vi "checkout.vi"(0 "HGF_Reference":refnum<class "HGF_Reference.lvclass">, 3 "timeout in ms (-1)":i32=-1, 5 "error in (no error)":errorcluster) -> (14 "dup HGF_Reference":refnum<class "HGF_Reference.lvclass">, 16 "Object":refnum<class>, 17 "got object?":bool, 19 "error out":errorcluster)   [LabVIEW 2014, in "HGF_BaseClasses.lvlib" / "HGF_Reference.lvclass"]
doc: "Check out the referenced Object.\n\n<B>Attention:</B> Error in is ignored, but forwarded.\nDo not forget to check in again, if you have got the object."
uses:
  HGF_Reference.lvclass
  HGF_Reference.lvclass/HGF_Reference.ctl
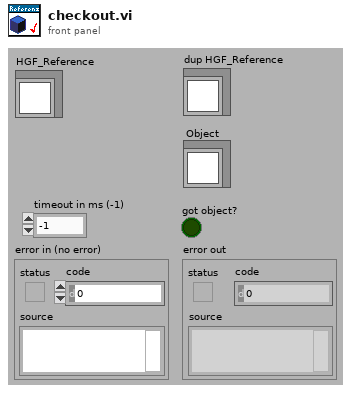
[diagram p1: front panel]
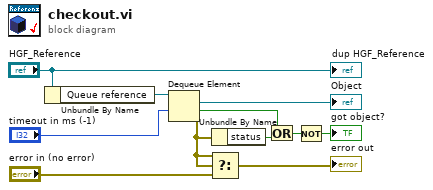
[diagram p0: block diagram]
diagram:
  n1 = Unbundle By Name("HGF_Reference") -> ("Queue reference"=w7:refnum<queue>)
  n2 = Dequeue Element(queue=w7, timeout in ms (-1)="timeout in ms (-1)") -> (element=→"Object":refnum<class>, timed out?=w10:bool, error out=w8:errorcluster)  [unwired: 1 in, 1 out]
  n3 = Select(t=w8, s=w8, f="error in (no error)") -> (s? t:f=→"error out":errorcluster)
  n4 = Unbundle By Name(w8) -> ("status"=w9:bool)
  n5 = Or(x=w10, y=w9) -> (x .or. y?=w11:bool)
  n6 = Not(x=w11) -> (.not. x?=→"got object?":bool)
  "dup HGF_Reference" <- "HGF_Reference"
